vi "Initialise.vi"(8 "error in (no error)":errorcluster, 11 "TimedDirector in":refnum<class "TimedDirector.lvclass">) -> (0 "error out":errorcluster, 3 "TimedDirector out":refnum<class "TimedDirector.lvclass">)   [LabVIEW 2023, in "HAF.lvlib" / "TimedDirector.lvclass"]
doc: "Initialises the Timed Director by storing the current millisecond count."
uses:
  TimedDirector.lvclass
  TimedDirector.lvclass/TimedDirector.ctl
  CommandDirector/CommandDirector.lvclass
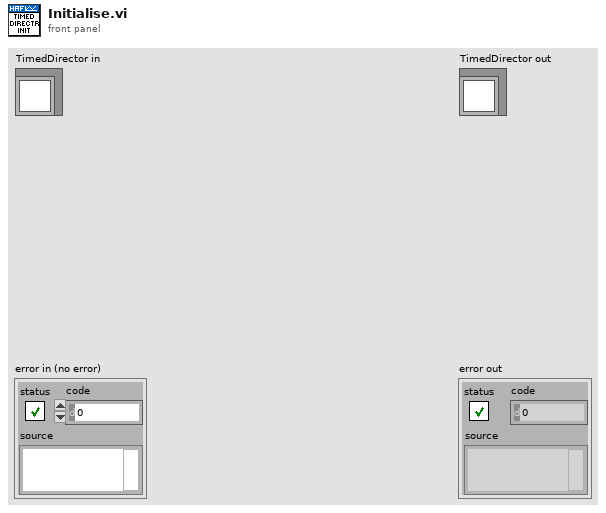
[diagram p1: front panel]
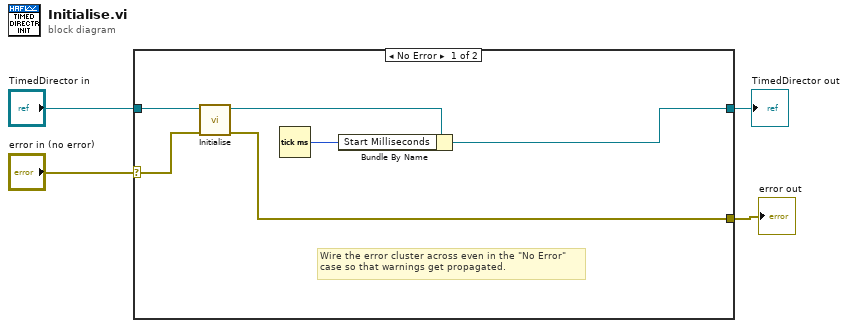
[diagram p0: block diagram]
diagram:
  n1 = case shown="No Error" "error in (no error)" {
    selector: "error in (no error)" -> [w9 w12]
    tunnel: [w5 w12] -> w3
    tunnel: [w6 w11] -> w1
    tunnel: "TimedDirector in" -> [w10 w11]
    frame No Error {
      # "Wire the error cluster across even in the \"No Error\"\ncase so that warnings get propagated."
      n2 = call-parent "Initialise.vi"("error in (no error)"=w9, "CommandDirector in"=w10) -> ("error out"=w5:errorcluster, "CommandDirector out"=w8:refnum<class "TimedDirector.lvclass">)  [unwired: 8 in]
      n3 = Tick Count (ms)() -> (millisecond timer value=w7:u32)
      n4 = Bundle By Name(cluster=w8, "Start Milliseconds"=w7) -> (w6:refnum<class "TimedDirector.lvclass">)
    }
    frame Error {
    }
  }
  "error out" <- w3
  "TimedDirector out" <- w1
